vi "riffle_index.vi"(2 "n catch":u16 step=1, 3 "n stim":u16 step=1, 4 "stim array in":u8[](array[numeric])) -> (0 "stim array out":u8[](array[numeric]), 1 "riffled index":i32)   [LabVIEW 2016]
uses:
  <vilib>/Analysis/1siggen.llb/Riffle Array (I32).vi
  <vilib>/Analysis/NI_AALBase.lvlib
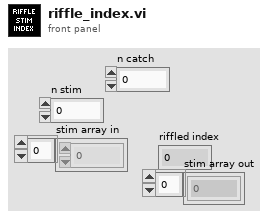
[diagram p1: front panel]
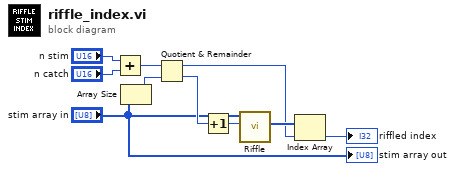
[diagram p0: block diagram]
diagram:
  n1 = Add(x="n stim", y="n catch") -> (x+y=w3:u16)
  n2 = Array Size(array="stim array in") -> (size(s)=w2:i32)
  n3 = Quotient & Remainder(x=w3, y=w2) -> (x-y*floor(x/y)=w6:i32, floor(x/y)=w10:i32)
  n4 = Increment(x=w10) -> (x+1=w9:i32)
  n5 = call-poly <vilib>:"Riffle.vi"("seed"=w9, "X"="stim array in") -> ("Riffled Index"=w8:i32[])  [unwired: 7 in, 2 out]
  n6 = Index Array(array=w8, index=w6) -> (element=→"riffled index":i32)
  "stim array out" <- "stim array in"
